vi "End Configuration.vi"(8 "error in (no error)":errorcluster, 10 "GPIB Espectrometro":refnum<visa-resource-name>="GPIB0::9::INSTR") -> (0 "error out":errorcluster)   [LabVIEW 2020]
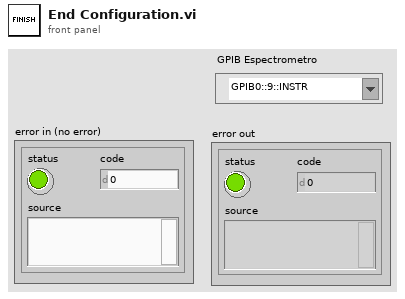
[diagram p1: front panel]
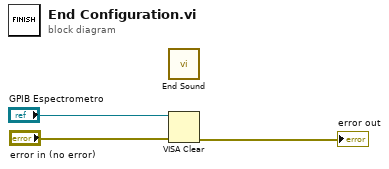
[diagram p0: block diagram]
diagram:
  n1 = call "End Sound.vi"() -> ()  [unwired: 12 in]
  n2 = VISA Clear(VISA resource name="GPIB Espectrometro", error in (no error)="error in (no error)") -> (error out=→"error out":errorcluster)  [unwired: 1 out]
